vi "VI Linearisierung v2.vi"() -> ()   [LabVIEW 2020, in "Linearisierung v2.lvlib"] (continued)
                        n1066 = Concatenate Strings(w1663, "\r", w1659) -> (w1662:string)
                        n1067 = local write "Status kalibrieren"(w1662) -> ()
                      }
                    }
                  }
                  frame #1 {
                    n1068 = call "FGV-Funktionstasten.vi"("Herkunft"="Linearisierung", "Zustand"=Zustaende."Cal-Gas", "Aktion"=Funktionstasten-Aktion."Zustand setzen") -> ()  [unwired: 5 in, 8 out]
                  }
                  frame #2 {
                    n1069 = call "FID Manuell Kalibrieren.vi"("Kalibrieren"=FID_Kalibrieren."THC Nullpunkt") -> ()  [unwired: 9 in, 2 out]
                  }
                  frame #3 {
                    n1070 = call "Gasteiler_Standby.vi"() -> ()  [unwired: 12 in]
                    n1071 = call "FGV-Funktionstasten.vi"("Herkunft"="Linearisierung", "Zustand"=Zustaende."Standby", "Aktion"=Funktionstasten-Aktion."Zustand setzen") -> ()  [unwired: 5 in, 8 out]
                  }
                }
              }
              frame "PNS" {
                n1072 = flat-sequence {
                  frame #0 {
                    n1073 = call "FGV-Funktionstasten.vi"("Herkunft"="Linearisierung", "Zustand"=Zustaende."Cal-Gas", "Aktion"=Funktionstasten-Aktion."Zustand setzen") -> ()  [unwired: 5 in, 8 out]
                  }
                  frame #1 {
                    n1074 = call "FID Manuell Kalibrieren.vi"("Kalibrieren"=FID_Kalibrieren."THC Nullpunkt") -> ()  [unwired: 9 in, 2 out]
                  }
                  frame #2 {
                    n1075 = call "FGV-Funktionstasten.vi"("Herkunft"="Linearisierung", "Zustand"=Zustaende."Standby", "Aktion"=Funktionstasten-Aktion."Zustand setzen") -> ()  [unwired: 5 in, 8 out]
                  }
                }
              }
              frame "ohne Gasteiler" {
                n1076 = flat-sequence {
                  frame #0 {
                    n1077 = call "FGV-Funktionstasten.vi"("Herkunft"="Linearisierung", "Zustand"=Zustaende."0-Gas", "Aktion"=Funktionstasten-Aktion."Zustand setzen") -> ()  [unwired: 5 in, 8 out]
                  }
                  frame #1 {
                    n1078 = call "FID Manuell Kalibrieren.vi"("Kalibrieren"=FID_Kalibrieren."THC Nullpunkt") -> ()  [unwired: 9 in, 2 out]
                  }
                  frame #2 {
                    n1079 = call "FGV-Funktionstasten.vi"("Herkunft"="Linearisierung", "Zustand"=Zustaende."Standby", "Aktion"=Funktionstasten-Aktion."Zustand setzen") -> ()  [unwired: 5 in, 8 out]
                  }
                }
              }
            }
          }
        }
        n1080 = case shown="True" "PMD  E kalibrieren" {
          tunnel: w1568 -> [_ w1575]
          tunnel: w1567 -> [_ w1574]
          frame False {
          }
          frame True {
            n1081 = case shown="\"Gasteiler\", Standard" w1575 {
              tunnel: w1574 -> [w1576 _ _]
              frame "Gasteiler", Default {
                n1082 = stacked-sequence {
                  tunnel: w1576 -> [w1577 _ _ _]
                  frame #0 {
                    n1083 = local read "Anforderung"() -> (w1578:T4)
                    n1084 = case shown="False" w1578 {
                      tunnel: w1577 -> [w1579 _]
                      frame False {
                        n1085 = local read "Status kalibrieren"() -> (w1582:string)
                        n1086 = call "Texte in VIs uebersetzen.vi"("Sprachliste"=w1579, "String zum Übersetzen"="Keine Anforderung Gasteiler!\n0-Gas manuell aufschalten!" ("String")) -> ("String zum Übersetzen"=w1580:string)  [unwired: 9 in, 4 out]
                        n1087 = Concatenate Strings(w1582, "\r", w1580) -> (w1583:string)
                        n1088 = local write "Status kalibrieren"(w1583) -> ()
                      }
                      frame True {
                        n1089 = call "Gasteiler_Endpunkt.vi"() -> ()  [unwired: 12 in]
                      }
                    }
                  }
                  frame #1 {
                    n1090 = call "FGV-Funktionstasten.vi"("Herkunft"="Linearisierung", "Zustand"=Zustaende."Cal-Gas", "Aktion"=Funktionstasten-Aktion."Zustand setzen") -> ()  [unwired: 5 in, 8 out]
                  }
                  frame #2 {
                    n1091 = call "PMA Manuell Kalibrieren.vi"("GT"=TRUE, "Kalibrieren"=Kalibrierung_O2."Endpunkt O2") -> ()  [unwired: 8 in, 2 out]
                  }
                  frame #3 {
                    n1092 = call "Gasteiler_Standby.vi"() -> ()  [unwired: 12 in]
                    n1093 = call "FGV-Funktionstasten.vi"("Herkunft"="Linearisierung", "Zustand"=Zustaende."Standby", "Aktion"=Funktionstasten-Aktion."Zustand setzen") -> ()  [unwired: 5 in, 8 out]
                  }
                }
              }
              frame "PNS" {
                n1094 = flat-sequence {
                  frame #0 {
                    n1095 = call "FGV-Funktionstasten.vi"("Herkunft"="Linearisierung", "Zustand"=Zustaende."Cal-Gas", "Aktion"=Funktionstasten-Aktion."Zustand setzen") -> ()  [unwired: 5 in, 8 out]
                  }
                  frame #1 {
                    n1096 = call "PMA Manuell Kalibrieren.vi"("Kalibrieren"=Kalibrierung_O2."Endpunkt O2") -> ()  [unwired: 9 in, 2 out]
                  }
                  frame #2 {
                    n1097 = call "FGV-Funktionstasten.vi"("Herkunft"="Linearisierung", "Zustand"=Zustaende."Standby", "Aktion"=Funktionstasten-Aktion."Zustand setzen") -> ()  [unwired: 5 in, 8 out]
                  }
                }
              }
              frame "ohne Gasteiler" {
                n1098 = flat-sequence {
                  frame #0 {
                    n1099 = call "FGV-Funktionstasten.vi"("Herkunft"="Linearisierung", "Zustand"=Zustaende."0-Gas", "Aktion"=Funktionstasten-Aktion."Zustand setzen") -> ()  [unwired: 5 in, 8 out]
                  }
                  frame #1 {
                    n1100 = call "PMA Manuell Kalibrieren.vi"("GT"=TRUE, "Kalibrieren"=Kalibrierung_O2."Endpunkt O2") -> ()  [unwired: 8 in, 2 out]
                  }
                  frame #2 {
                    n1101 = call "FGV-Funktionstasten.vi"("Herkunft"="Linearisierung", "Zustand"=Zustaende."Standby", "Aktion"=Funktionstasten-Aktion."Zustand setzen") -> ()  [unwired: 5 in, 8 out]
                  }
                }
              }
            }
          }
        }
      }
      event Value Change {
        n1102 = event-data() -> ()  [unwired: 1 in, 1 out]
        n1103 = call "FGV CalGas.vi"("Aktionen"=FGV_CalGas_Aktionen."Aufschaltung CalGas", "Aufschaltung CalGas"="Aufschaltung CalGas") -> ()  [unwired: 5 in, 5 out]
      }
      event Value Change {
        w1724 = T4 TRUE  # Gasteiler Spülen
        n1104 = event-data() -> ()  [unwired: 1 in, 1 out]
        n1105 = case shown="True" "Gasteiler Spülen" {
          frame False {
          }
          frame True {
            n1106 = call "FGV Gasteiler.vi"("Aktionen"=Aktionen_FGV_Gasteiler_Daten."lesen") -> ("Gasteiler Type"=w1736:T15)  [unwired: 11 in, 7 out]
            n1107 = case shown="0, Standard" w1736 {
              frame 0, Default {
                n1108 = call "AK Komm.vi"("Aktionen"=Aktionen_AK_Komm."SRUC") -> ()  [unwired: 4 in, 7 out]
              }
            }
          }
        }
        n1109 = case shown="True" "Gasteiler EP spülen" {
          frame False {
          }
          frame True {
            n1110 = call "FGV Gasteiler.vi"("Aktionen"=Aktionen_FGV_Gasteiler_Daten."lesen") -> ("Gasteiler Type"=w1727:T15)  [unwired: 11 in, 7 out]
            n1111 = case shown="1" w1727 {
              frame 1 {
                w1729 = u32 750 ("Zu wartende ms")
                n1112 = flat-sequence {
                  tunnel: w1729 -> [w1731]
                  tunnel: w1729 -> [w1733]
                  frame #0 {
                    n1113 = call "AK Komm_ALT.vi"("Aktionen_ALT"=Aktionen_AK_Komm_ALT."SSPL") -> ()  [unwired: 6 in, 5 out]
                  }
                  frame #1 {
                    n1114 = Wait (ms)(milliseconds to wait=w1731) -> ()  [unwired: 1 out]
                  }
                  frame #2 {
                    n1115 = call "AK Komm_ALT.vi"("Aktionen_ALT"=Aktionen_AK_Komm_ALT."SSPL") -> ()  [unwired: 6 in, 5 out]
                  }
                  frame #3 {
                    n1116 = Wait (ms)(milliseconds to wait=w1733) -> ()  [unwired: 1 out]
                  }
                  frame #4 {
                    n1117 = call "AK Komm_ALT.vi"("Aktionen_ALT"=Aktionen_AK_Komm_ALT."SSPL") -> ()  [unwired: 6 in, 5 out]
                  }
                }
              }
              frame 0, Default {
                n1118 = call "AK Komm.vi"("Aktionen"=Aktionen_AK_Komm."SSPL") -> ()  [unwired: 4 in, 7 out]
              }
            }
          }
        }
      }
      event Value Change {
        n1119 = event-data() -> ()  [unwired: 1 in, 1 out]
        n1120 = call "FGV Gasteiler.vi"("Aktionen"=Aktionen_FGV_Gasteiler_Daten."lesen") -> ("Anforderung"=w1743:bool)  [unwired: 11 in, 7 out]
        n1121 = case shown="True" w1743 {
          tunnel: w1742 -> [w1745 _]
          frame False {
            n1122 = call "Texte in VIs uebersetzen.vi"("Sprachliste"=w1745, "String zum Übersetzen"="Gasteiler\nKeine Anforderung!" ("Nachricht")) -> ("String zum Übersetzen"=w1748:string)  [unwired: 9 in, 4 out]
            n1123 = call "Texte in VIs uebersetzen.vi"("Sprachliste"=w1745, "String zum Übersetzen"="OK") -> ("String zum Übersetzen"=w1747:string)  [unwired: 9 in, 4 out]
            n1124 = One Button Dialog(message=w1748, button name ("OK")=w1747) -> ()  [unwired: 1 out]
          }
          frame True {
            n1125 = call "FGV_Betreibsdaten.vi"("Gase schreiben"="Gase", "Enum"=Aktion_FGV_Betriebsdaten."Gase schreiben") -> ("error out"=w1760:errorcluster)  [unwired: 10 in, 7 out]
            n1126 = call "FGV_Kommunikation.vi"("error in"=w1760, "Aktion"=Aktion_FGV_Kom."Gase") -> ("error out"=w1756:errorcluster)  [unwired: 5 in, 4 out]
            n1127 = call "FGV_Betreibsdaten.vi"("error in (no error)"=w1756, "Enum"=Aktion_FGV_Betriebsdaten."Lesen") -> ("Gase schreiben"=w1755:T63, "Gase lesen"=w1754:T63, "error out"=w1752:errorcluster)  [unwired: 10 in, 5 out]
            n1128 = Not Equal?(x=w1755, y=w1754) -> (x != y?=w1757:T181)
            n1129 = Cluster To Array(cluster=w1757) -> (array=w1758:bool[])
            n1130 = call <vilib>:"Clear Errors.vi"("error in (no error)"=w1752) -> ()  [unwired: 5 in, 2 out]
            n1131 = Or Array Elements(Boolean array=w1758) -> (logical OR=→"Fehler Kommunikation\nGase":bool)
          }
        }
      }
      event "Vaporizer einschalten": Value Change {
        n1132 = event-data() -> ()  [unwired: 1 in, 1 out]
        n1133 = call "FGV Gasteiler.vi"("Aktionen"=Aktionen_FGV_Gasteiler_Daten."lesen") -> ("Anforderung"=w1766:bool)  [unwired: 11 in, 7 out]
        n1134 = case shown="True" w1766 {
          tunnel: w1765 -> [w1768 _]
          frame False {
            n1135 = call "Texte in VIs uebersetzen.vi"("Sprachliste"=w1768, "String zum Übersetzen"="Gasteiler\nKeine Anforderung!" ("Nachricht")) -> ("String zum Übersetzen"=w1771:string)  [unwired: 9 in, 4 out]
            n1136 = call "Texte in VIs uebersetzen.vi"("Sprachliste"=w1768, "String zum Übersetzen"="OK") -> ("String zum Übersetzen"=w1770:string)  [unwired: 9 in, 4 out]
            n1137 = One Button Dialog(message=w1771, button name ("OK")=w1770) -> ()  [unwired: 1 out]
          }
          frame True {
            n1138 = case shown="True" "Vaporizer einschalten" {
              tunnel: [w1787 w1794] -> w1778
              frame False {
                n1139 = property on="Pumpe Ein/Aus" class="Ring (strikt)"("Value"=0.0 ("Wert")) -> (error out=w1789:errorcluster)  [unwired: 2 in, 1 out]
                n1140 = property on="Solltemperatur" class="DigWert (strikt)"("Value"=0.0 ("Wert")) -> (error out=w1788:errorcluster)  [unwired: 2 in, 1 out]
                n1141 = property on="Vaporizer" class="Cluster (strikt)"("DisabledEnum"=T66."Disabled and Grayed Out" ("Deaktiviert")) -> (error out=w1790:errorcluster)  [unwired: 2 in, 1 out]
                n1142 = Merge Errors(w1790, w1789, w1788) -> (w1787:errorcluster)
              }
              frame True {
                n1143 = property on="Wasser / Reagent" class="Ring (strikt)"() -> (error out=w1797:errorcluster, "Value"=w1798:dbl)  [unwired: 2 in, 1 out]
                n1144 = case shown="0, Standard" w1798 {
                  tunnel: [w1801 w1804] -> w1796
                  tunnel: w1797 -> [w1800 w1803]
                  frame 0, Default {
                    n1145 = property on="Reagent" class="Ring (strikt)"(error in=w1800, "DisabledEnum"=T66."Disabled and Grayed Out" ("Deaktiviert")) -> (error out=w1801:errorcluster)  [unwired: 1 in, 1 out]
                  }
                  frame 1 {
                    n1146 = property on="Reagent" class="Ring (strikt)"(error in=w1803, "DisabledEnum"=T66."Enabled" ("Deaktiviert")) -> (error out=w1804:errorcluster)  [unwired: 1 in, 1 out]
                  }
                }
                n1147 = property on="Vaporizer" class="Cluster (strikt)"("DisabledEnum"=T66."Enabled" ("Deaktiviert")) -> (error out=w1795:errorcluster)  [unwired: 2 in, 1 out]
                n1148 = Merge Errors(w1795, w1796) -> (w1794:errorcluster)
              }
            }
            n1149 = call "FGV_Vaporizer.vi"("Enum"=T148."Vaporizer schreiben", "error in (no error)"=w1778, "Vaporizer schreiben"="Vaporizer") -> ("error out"=w1777:errorcluster)  [unwired: 5 in, 3 out]
            n1150 = call "FGV_Kommunikation.vi"("error in"=w1777, "Aktion"=Aktion_FGV_Kom."Vaporizer" ("Enum")) -> ("error out"=w1784:errorcluster)  [unwired: 5 in, 4 out]
            n1151 = call "FGV_Vaporizer.vi"("Enum"=T148."Lesen", "error in (no error)"=w1784) -> ("error out"=w1773:errorcluster, "Vaporizer_schreiben"=w1780:T65, "Vaporizer_lesen"=w1781:T65)  [unwired: 6 in, 1 out]
            n1152 = Not Equal?(x=w1781, y=w1780) -> (x != y?=w1782:T182)
            n1153 = Cluster To Array(cluster=w1782) -> (array=w1783:bool[])
            n1154 = call <vilib>:"Clear Errors.vi"("error in (no error)"=w1773) -> ()  [unwired: 5 in, 2 out]
            n1155 = Or Array Elements(Boolean array=w1783) -> (logical OR=→"Fehler Kommunikation\nVaporizer":bool)
          }
        }
      }
      event "Standartwerte Hovacal": Value Change {
        n1156 = event-data() -> ()  [unwired: 1 in, 1 out]
        n1157 = call "FGV Gasteiler.vi"("Aktionen"=Aktionen_FGV_Gasteiler_Daten."lesen") -> ("Anforderung"=w1810:bool)  [unwired: 11 in, 7 out]
        n1158 = case shown="True" w1810 {
          tunnel: w1809 -> [w1812 _]
          frame False {
            n1159 = call "Texte in VIs uebersetzen.vi"("Sprachliste"=w1812, "String zum Übersetzen"="Gasteiler\nKeine Anforderung!" ("Nachricht")) -> ("String zum Übersetzen"=w1815:string)  [unwired: 9 in, 4 out]
            n1160 = call "Texte in VIs uebersetzen.vi"("Sprachliste"=w1812, "String zum Übersetzen"="OK") -> ("String zum Übersetzen"=w1814:string)  [unwired: 9 in, 4 out]
            n1161 = One Button Dialog(message=w1815, button name ("OK")=w1814) -> ()  [unwired: 1 out]
          }
          frame True {
            n1162 = case shown="True" "Standartwerte Hovacal" {
              tunnel: [w1838 w1843] -> w1825
              frame True {
                w1834 = 0.0 ("Wert")
                w1832 = T66."Disabled and Grayed Out" ("Deaktiviert")
                n1163 = property on="Gesamtdurchfluss" class="DigWert (strikt)"("DisabledEnum"=w1832, "Value"=3.0 ("Wert")) -> (error out=w1837:errorcluster)  [unwired: 2 in, 1 out]
                n1164 = property on="Ausgangskonzentration\nKomponente 2" class="DigWert (strikt)"("DisabledEnum"=w1832, "Value"=w1834) -> (error out=w1835:errorcluster)  [unwired: 2 in, 1 out]
                n1165 = property on="Eingangskonzentration \nKomponente 2" class="DigWert (strikt)"("DisabledEnum"=w1832, "Value"=w1834) -> (error out=w1836:errorcluster)  [unwired: 2 in, 1 out]
                n1166 = property on="Eingangskonzentration \nTrägergas" class="DigWert (strikt)"("DisabledEnum"=w1832, "Value"=100.0 ("Wert")) -> ()  [unwired: 2 in, 2 out]
                n1167 = Merge Errors(w1837, w1836, w1835) -> (w1838:errorcluster)
              }
              frame False {
                w1839 = T66."Enabled" ("Deaktiviert")
                n1168 = property on="Gesamtdurchfluss" class="DigWert (strikt)"("DisabledEnum"=w1839) -> (error out=w1842:errorcluster)  [unwired: 2 in, 1 out]
                n1169 = property on="Eingangskonzentration \nKomponente 2" class="DigWert (strikt)"("DisabledEnum"=w1839) -> (error out=w1841:errorcluster)  [unwired: 2 in, 1 out]
                n1170 = property on="Ausgangskonzentration\nKomponente 2" class="DigWert (strikt)"("DisabledEnum"=w1839) -> (error out=w1840:errorcluster)  [unwired: 2 in, 1 out]
                n1171 = Merge Errors(w1842, w1841, w1840) -> (w1843:errorcluster)
              }
            }
            n1172 = call "FGV_Betreibsdaten.vi"("Sollwert schreiben"="Daten", "error in (no error)"=w1825, "Enum"=Aktion_FGV_Betriebsdaten."Sollwerte schreiben" ("Aktion")) -> ("error out"=w1824:errorcluster)  [unwired: 9 in, 7 out]
            n1173 = call "FGV_Kommunikation.vi"("error in"=w1824, "Aktion"=Aktion_FGV_Kom."Betriebsparameter" ("Enum")) -> ("error out"=w1821:errorcluster)  [unwired: 5 in, 4 out]
            n1174 = call "FGV_Betreibsdaten.vi"("error in (no error)"=w1821, "Enum"=Aktion_FGV_Betriebsdaten."Lesen" ("Aktion")) -> ("Sollwerte lesen"=w1829:T64, "Sollwert für Vergleich"=w1828:T64, "error out"=w1819:errorcluster)  [unwired: 10 in, 5 out]
            n1175 = Not Equal?(x=w1829, y=w1828) -> (x != y?=w1826:T183)
            n1176 = call <vilib>:"Clear Errors.vi"("error in (no error)"=w1819) -> ()  [unwired: 5 in, 2 out]
            n1177 = Cluster To Array(cluster=w1826) -> (array=w1827:bool[])
            n1178 = Or Array Elements(Boolean array=w1827) -> (logical OR=→"Fehler Kommunikaton\nBetriebsdaten":bool)
          }
        }
      }
      event Value Change {
        n1179 = event-data() -> ()  [unwired: 1 in, 1 out]
        n1180 = call "Genauigkeit Polynom 2 String.vi"() -> ("Format-String Polynom 2 Sting"=w1845:string)  [unwired: 9 in, 2 out]
        n1181 = for {
          tunnel: "PolynomTabelleEingabe" -> [w1856] mode=indexing
          tunnel: [w1855] -> w1847 mode=indexing
          tunnel: w1845 -> [w1854]
          # "#PolynomDBL"
          n1182 = for {
            tunnel: w1856 -> [w1860] mode=indexing
            tunnel: [w1859] -> w1855 mode=indexing
            tunnel: w1854 -> [w1857]
            n1183 = Scan Value(string=w1860, format string=w1857, default (0 dbl)=0.0) -> (value=w1859:dbl)  [unwired: 1 out]
          }
        }
        n1184 = call "Polynom Daten speichern.vi"("Aktionen"=Aktionen_Polynom_Daten_speichern."schreiben alle", "Aktiv"="PolynomAktiv", "Polynome"=w1847) -> ("Polynome"=w1853:dbl[][])  [unwired: 3 in, 5 out]
        n1185 = call "Polynom Daten speichern.vi"("Aktionen"=Aktionen_Polynom_Daten_speichern."speichern", "Polynome"=w1853) -> ()  [unwired: 4 in, 6 out]
      }
      event "Hauptregisterkarte": Value Change {
        n1186 = event-data() -> ()  [unwired: 1 in, 1 out]
        n1187 = call "Komponentenausgabe.vi"() -> ("Gaskomponente"=w1865:T7)  [unwired: 8 in, 3 out]
        n1188 = call "Einheiten finden.vi"("Komponente"=w1865) -> ("Einheit in String"=w1864:string)  [unwired: 6 in, 4 out]
        n1189 = case shown="\"LIN Anpassung\"" "Hauptregisterkarte" {
          tunnel: w1865 -> [_ _ w1918 w1966 _ _ _ _ _ _]
          tunnel: [_ _ _ _ _ _ _ TRUE _ _] -> w1869
          tunnel: w1868 -> [_ w1887 _ _ _ _ _ _ _ _]
          tunnel: w1864 -> [_ _ w1928 w1985 _ _ _ _ _ _]
          tunnel: w1867 -> [_ _ _ w1986 _ _ _ _ _ _]
          tunnel: w1866 -> [_ w1886 w1927 _ _ _ _ _ _ _]
          tunnel: w1862 -> [_ _ _ _ _ _ _ _ _ w2030]
          tunnel: w1861 -> [_ _ _ _ _ _ _ _ _ w2029]
          frame "Einstellungen", Default {
          }
          frame "Daten aufzeichnen" {
            # "#LinEinheiten #HovaCALMultiMFC"
            n1190 = local read "passive Komponente:"() -> (w1882:u16)
            n1191 = local read "Gasnummer Generieren"() -> (w1874:T49)
            n1192 = Equal To 0?(x=w1882) -> (x = 0?=w1884:bool)
            n1193 = Decrement(x=w1882) -> (x-1=w1883:u16)
            n1194 = call "Komponentenausgabe HovaCAL fix.vi"("Gasnummer in"=w1874) -> ("Gaskomponente"=w1880:T7)  [unwired: 7 in, 3 out]
            n1195 = Select(t=w1880, s=w1884, f=w1883) -> (s? t:f=w1879:T7)
            n1196 = call "Einheiten finden.vi"("Komponente"=w1879) -> ("Einheit in String"=w1881:string)  [unwired: 6 in, 4 out]
            n1197 = call "Lin Daten aufarbeiten.vi"("Index (Seite)"=w1879, "Aktionen"=Aktion_Lin_Daten_aufarbeiten."lesen") -> ("Eingabetabelle"=w1890:T54, "Lin-Polynom"=w1878:T119)  [unwired: 15 in, 9 out]
            n1198 = disable-structure shown="Aktiviert" {
              disable-tunnel: w1879 -> [w1895 w1900]
              disable-tunnel: w1878 -> [w1894 w1901]
              disable-tunnel: [w1893 w1903] -> w1877
              disable-tunnel: [w1892 w1902] -> w1876
              disable-tunnel: [_ w1904] -> w1875
              frame Disabled {
                n1199 = call "Get Autorange Bereiche.vi"("Gaskomponente"=w1895) -> ("error out"=w1896:errorcluster, "Autorange Bereiche"=w1899:T7[])  [unwired: 8 in, 1 out]
                n1200 = call "Set Spanfactors and Offests in Lin-Protocol.vi"("Lin-Polynom"=w1894) -> ("Offset"=w1897:sgl[], "Span"=w1898:sgl[])  [unwired: 7 in, 2 out]
                n1201 = call "Get Autorange Spanfactors and Offsets.vi"("error in (no error)"=w1896, "Autorange Bereiche"=w1899, "Offset"=w1897, "Span"=w1898) -> ("Autorange Offsets"=w1892:string, "Autorange Spanfactors"=w1893:string)  [unwired: 3 in, 3 out]
              }
              frame Enabled {
                # "#PDF_manu_MG"
                n1202 = call "Component Get Daten aufzeichnen.vi"("Lin-Polynom"=w1901, "Gaskomponente"=w1900) -> ("Autorange Offsets"=w1902:string, "Autorange Spanfactors"=w1903:string, "Polynome"=w1904:T184)  [unwired: 6 in, 1 out]
              }
            }
            n1203 = call "Einheiten in Tabellenspalten.vi"("Einheit"=w1881, "Tabelle (Eingang)"=w1887) -> ("Einheit out"=w1885:string)  [unwired: 7 in, 2 out]
            n1204 = local write "Einheit"(w1881) -> ()
            n1205 = local write "Einheit Deviation"(w1881) -> ()
            n1206 = call "AusgabeTabelle zusammenbauen.vi"("Eingabetabelle"=w1890) -> ("Eingabetabelle behandelt"=w1888:string[][], "Ausgabetabelle"=→"Ausgabetabelle":T53)  [unwired: 8 in, 1 out]
            n1207 = call "Einheiten in Tabellenspalten.vi"("Einheit"=w1885, "Tabelle (Eingang)"=w1886) -> ()  [unwired: 7 in, 3 out]
            n1208 = local write "Eingabetabelle"(w1888) -> ()
            n1209 = local write "Polynom"(w1875) -> ()
            n1210 = local write "Spanfactor"(w1877) -> ()
            n1211 = local write "Offset"(w1876) -> ()
          }
          frame "EPA 1065-307" {
            # "#PDF_manu_MG"
            # "#LinEinheiten"
            n1212 = local read "Gasnummer EPA"() -> (w1925:T49)
            n1213 = call "Einheiten in Tabellenspalten.vi"("Einheit"=w1928, "Tabelle (Eingang)"=w1927) -> ()  [unwired: 7 in, 3 out]
            n1214 = call "aktueller SPAN und Komponent Index.vi"() -> ("akt SPAN out"=w1913:i32)  [unwired: 7 in, 4 out]
            n1215 = Decrement(x=w1925) -> (x-1=w1909:T49)
            n1216 = local read "EPA Filename override"() -> (w1907:T1)
            n1217 = Bundle("akt SPAN out"=w1913, w1909) -> (w1912:cluster{"akt SPAN out":i32, T49})  [unwired: 1 in]
            n1218 = call "EPA Polynom Ordnung je Komponente für Protokoll.vi"("Aktion"=Aktion_EPA_Polynom_Ordnung_je_Komponente_für_Protokoll."lesen", "Index in"=w1912) -> ("EPA Optionsfeld out"=w1914:T2)  [unwired: 5 in, 3 out]
            n1219 = call "Lin Daten aufarbeiten.vi"("Index (Seite)"=w1918, "Aktionen"=Aktion_Lin_Daten_aufarbeiten."lesen") -> ("Index (Seite) out"=w1921:i32, "Lin-Polynom"=w1919:T119, "error out"=w1920:errorcluster)  [unwired: 15 in, 8 out]
            n1220 = Bundle By Name(cluster=w1919, "EPA Optionsfeld"=w1914) -> (w1923:T119)
            n1221 = call "FGV SPAN Verriegelung.vi"("aktion"=Aktion_FGV_SPAN_Verriegelung."lesen") -> ("locked"=w1910:bool)  [unwired: 8 in, 2 out]
            n1222 = local write "EPA Optionsfeld"(w1914) -> ()
            n1223 = Not(x=w1907) -> (.not. x?=w1906:T1)
            n1224 = Not(x=w1910) -> (.not. x?=w1905:bool)
            n1225 = call "Lin Daten aufarbeiten.vi"("Index (Seite)"=w1921, "Lin-Polynom"=w1923, "error in (no error)"=w1920, "Aktionen"=Aktion_Lin_Daten_aufarbeiten."Protkolldaten") -> ("Index (Seite) out"=w1917:i32, "error out"=w1915:errorcluster)  [unwired: 13 in, 9 out]
            n1226 = And(x=w1906, y=w1905) -> (x .and. y?=w1908:T1)
            n1227 = case shown="True" w1908 {
              tunnel: w1917 -> [_ w1944]
              tunnel: w1909 -> [_ w1943]
              frame False {
              }
              frame True {
                # "#Lin_Load_Polynom_Question"
                n1228 = disable-structure shown="Aktiviert" {
                  disable-tunnel: [w1949 w1955] -> w1946
                  disable-tunnel: [w1948 w1954] -> w1945
                  disable-tunnel: w1944 -> [w1947 _]
                  disable-tunnel: w1943 -> [_ w1953]
                  frame Disabled {
                    n1229 = call "FGV Gasliste.vi"("Aktionen"=FGV_FT-IR_Gasliste_Aktionen."lesen") -> ("Aktuelle Gasliste gesamt"=w1951:T48[])  [unwired: 8 in, 2 out]
                    n1230 = Index Array(array=w1951, index=w1947) -> (element=w1950:T48)
                    n1231 = call "Namen fuer File erzeugen.vi"("String Eingabe"=w1950) -> ("File Name LIN"=w1948:string, "File Name EPA"=w1949:string)  [unwired: 9 in]
                  }
                  frame Enabled {
                    n1232 = call "MG FileName.vi"("Gasnummer:"=w1953) -> ("LIN TXT Datei Name"=w1954:string, "EPA TXT Datei Name"=w1955:string)  [unwired: 7 in, 2 out]
                  }
                }
                n1233 = local write "EPA Filename"(w1946) -> ()
                n1234 = local write "File Name LIN"(w1945) -> ()
              }
            }
            n1235 = control-ref of="EPA Auswertung"() -> (w1929:refnum<vi>)
            n1236 = call "Lin Daten aufarbeiten.vi"("Index (Seite)"=w1917, "error in (no error)"=w1915, "Aktionen"=Aktion_Lin_Daten_aufarbeiten."EPA auswerten") -> ("Index (Seite) out"=w1916:i32, "error out"=w1940:errorcluster)  [unwired: 14 in, 9 out]
            n1237 = call "Lin Daten aufarbeiten.vi"("Index (Seite)"=w1916, "error in (no error)"=w1940, "Aktionen"=Aktion_Lin_Daten_aufarbeiten."lesen") -> ("Aktiv EPA"=w1932:T57, "Eingabetabelle"=w1937:T54, "EPA Auswertung"=w1931:cluster{sgl[], sgl[], bool[]}, "error out"=w1939:errorcluster)  [unwired: 14 in, 7 out]
            n1238 = call "EPA_Tabelle zusammenbauen.vi"("error in (no error)"=w1939, "Eingabetabelle"=w1937) -> ("error out"=w1935:errorcluster, "XY-Graph"=→"XY-Graph EPA":cluster{dbl[], dbl[]}[], "EPA Ausgabetabelle"=→"EPA Ausgabetabelle":string[][])  [unwired: 7 in]
            n1239 = local write "Aktiv"(w1932) -> ()
            n1240 = Unbundle(w1931) -> (w1930:bool[])  [unwired: 2 out]
            n1241 = call "FGV Auswertung sammeln.vi"("Aktion"=Aktion_FGV_Auswertung_sammeln."lesen", "error in (no error)"=w1935) -> ("LINVer Auswertung"=→"EPA Auswertung":string[][])  [unwired: 7 in, 2 out]
            n1242 = call "Zellen einfaerben.vi"("Färben"=w1930, "Tabellenref."=w1929) -> ()  [unwired: 10 in]
          }
          frame "LIN Anpassung" {
            # "#PDF_manu_MG"
            # "#LinEinheiten #AutorangeSpanfactorsOffsets"
            n1243 = local read "Gasnummer LIN"() -> (w1971:T49)
            n1244 = call "Einheiten in Tabellenspalten.vi"("Einheit"=w1985, "Tabelle (Eingang)"=w1986) -> ()  [unwired: 7 in, 3 out]
            n1245 = call "aktueller SPAN und Komponent Index.vi"() -> ("akt SPAN out"=w1967:i32)  [unwired: 7 in, 4 out]
            n1246 = Decrement(x=w1971) -> (x-1=w1960:T49)
            n1247 = Bundle("akt SPAN out"=w1967, w1960) -> (w1968:cluster{"akt SPAN out":i32, T49})  [unwired: 1 in]
            n1248 = local read "LIN Filename override"() -> (w1958:T1)
            n1249 = call "LIN Polynom Ordnung je Komponente für Protokoll.vi"("Aktion"=Aktion_LIN_Polynom_Ordnung_je_Komponente_für_Protokoll."lesen", "Index in"=w1968) -> ("Polynom-Ordnung view only out"=w1969:T55)  [unwired: 3 in, 6 out]
            n1250 = local write "Polynom-Ordnung"(w1969) -> ()
            n1251 = call "FGV SPAN Verriegelung.vi"("aktion"=Aktion_FGV_SPAN_Verriegelung."lesen") -> ("locked"=w1961:bool)  [unwired: 8 in, 2 out]
            n1252 = call "Lin Daten aufarbeiten.vi"("Index (Seite)"=w1966, "Polynom-Ordnung"=w1969, "Aktionen"=Aktion_Lin_Daten_aufarbeiten."Lin auswerten") -> ("Index (Seite) out"=w1964:i32, "error out"=w1987:errorcluster)  [unwired: 14 in, 9 out]
            n1253 = call "Get Autorange Bereiche.vi"("Gaskomponente"=w1966) -> ("error out"=w1977:errorcluster, "Autorange Bereiche"=w1984:T7[])  [unwired: 8 in, 1 out]
            n1254 = Not(x=w1961) -> (.not. x?=w1956:bool)
            n1255 = Not(x=w1958) -> (.not. x?=w1957:T1)
            n1256 = call "Lin Daten aufarbeiten.vi"("Index (Seite)"=w1964, "error in (no error)"=w1987, "Aktionen"=Aktion_Lin_Daten_aufarbeiten."lesen") -> ("Aktiv LIN"=w1989:bool[], "Eingabetabelle"=w1993:T54, "Index (Seite) out"=w1963:i32, "Lin-Polynom"=w1965:T119, "error out"=w1982:errorcluster)  [unwired: 14 in, 6 out]
            n1257 = And(x=w1957, y=w1956) -> (x .and. y?=w1959:T1)
            n1258 = call "Set Spanfactors and Offests in Lin-Protocol.vi"("error in (no error)"=w1982, "Lin-Polynom"=w1965) -> ("error out"=w1981:errorcluster, "Offset"=w1978:sgl[], "Span"=w1979:sgl[], "Lin-Polynom out"=w1980:T119)  [unwired: 6 in]
            n1259 = case shown="True" w1959 {
              tunnel: w1963 -> [_ w1995]
              tunnel: w1960 -> [_ w1994]
              frame False {
              }
              frame True {
                # "#Lin_Load_Polynom_Question"
                n1260 = disable-structure shown="Aktiviert" {
                  disable-tunnel: [w2000 w2006] -> w1997
                  disable-tunnel: [w1999 w2005] -> w1996
                  disable-tunnel: w1995 -> [w1998 _]
                  disable-tunnel: w1994 -> [_ w2004]
                  frame Disabled {
                    n1261 = call "FGV Gasliste.vi"("Aktionen"=FGV_FT-IR_Gasliste_Aktionen."lesen") -> ("Aktuelle Gasliste gesamt"=w2002:T48[])  [unwired: 8 in, 2 out]
                    n1262 = Index Array(array=w2002, index=w1998) -> (element=w2001:T48)
                    n1263 = call "Namen fuer File erzeugen.vi"("String Eingabe"=w2001) -> ("File Name LIN"=w1999:string, "File Name EPA"=w2000:string)  [unwired: 9 in]
                  }
                  frame Enabled {
                    n1264 = call "MG FileName.vi"("Gasnummer:"=w2004) -> ("LIN TXT Datei Name"=w2005:string, "EPA TXT Datei Name"=w2006:string)  [unwired: 7 in, 2 out]
                  }
                }
                n1265 = local write "EPA Filename"(w1997) -> ()
                n1266 = local write "File Name LIN"(w1996) -> ()
              }
            }
            n1267 = call "LinTabelle zusammenbauen.vi"("error in (no error)"=w1982, "Eingabetabelle"=w1993) -> ("XY-Graph"=→"XY-Graph LIN":cluster{dbl[], dbl[]}[], "LIN Ausgabetabelle"=→"LIN Ausgabetabelle":string[][])  [unwired: 6 in, 2 out]
            n1268 = call "Lin Daten aufarbeiten.vi"("Index (Seite)"=w1963, "Lin-Polynom"=w1980, "error in (no error)"=w1981, "Aktionen"=Aktion_Lin_Daten_aufarbeiten."Protkolldaten") -> ("Lin-Polynom"=w1974:T119)  [unwired: 13 in, 10 out]
            n1269 = local write "Aktiv LIN"(w1989) -> ()
            n1270 = Unbundle By Name(w1974) -> ("Polynomkoeff."=w1976:dbl[])
            n1271 = call "Get Autorange Spanfactors and Offsets.vi"("error in (no error)"=w1977, "Autorange Bereiche"=w1984, "Offset"=w1978, "Span"=w1979) -> ("Autorange Offsets"=w1972:string, "Autorange Spanfactors"=w1973:string)  [unwired: 3 in, 3 out]
            n1272 = Array To Cluster(array=w1976) -> (cluster=w1975:T185)
            n1273 = local write "LIN Polynomkoeffizienten"(w1975) -> ()
            n1274 = local write "Spanfactor LIN"(w1973) -> ()
            n1275 = local write "Offset LIN"(w1972) -> ()
          }
          frame "Polynomkoeffizienten" {
            n1276 = call "Polynom Daten speichern.vi"("Aktionen"=Aktionen_Polynom_Daten_speichern."lesen") -> ("Aktiv"=w2009:bool[], "Polynome"=w2008:dbl[][])  [unwired: 5 in, 4 out]
            n1277 = call "Genauigkeit Polynom 2 String.vi"() -> ("Format-String Polynom 2 Sting"=w2007:string)  [unwired: 9 in, 2 out]
            n1278 = for {
              tunnel: w2008 -> [w2014] mode=indexing
              tunnel: [w2013] -> w2010 mode=indexing
              tunnel: w2007 -> [w2012]
              # "#PolynomDBL"
              n1279 = for {
                tunnel: w2014 -> [w2017] mode=indexing
                tunnel: [w2016] -> w2013 mode=indexing
                tunnel: w2012 -> [w2015]
                n1280 = Format Value(format string=w2015, value (0)=w2017) -> (output string=w2016:string)  [unwired: 1 in]
              }
            }
            n1281 = local write "PolynomAktiv"(w2009) -> ()
            n1282 = local write "PolynomTabelleEingabe"(w2010) -> ()
          }
          frame "HovaCal Einstellungen" {
          }
          frame "HovaCAL Interface" {
            n1283 = call "FGV_HovaCAL_Interface_GetData.vi"("first flags in"=T151 {"first contact in"=TRUE, "first actual values in "=TRUE}, "Aktion"=Aktion_FGV_HovaCAL_Interface_GetData."first contact") -> ()  [unwired: 5 in, 5 out]
          }
          frame "Spanfaktor" {
            n1284 = call "Spantabellenanzeige.vi"() -> ("SpanTabelle"=w2022:T48[][])  [unwired: 10 in, 1 out]
            n1285 = Delete From Array(array=w2022, length=3 ("Länge"), index (col)=0 ("Deaktivierter Index (Spalte)")) -> (deleted portion=w2020:T48[][], array with subset deleted=w2021:T48[][])  [unwired: 1 in]
            n1286 = local write "SpanTabelleEingabe"(w2021) -> ()
            n1287 = local write "SpanTabelleAnzeige"(w2020) -> ()
          }
          frame "Kalibrierung" {
          }
          frame "Span Einstellungen" {
            n1288 = call "Span Register setzen.vi"("GD Span Eingänge"=w2030, "automatisch Boolesch (Eingang)"=w2029) -> ()  [unwired: 3 in, 7 out]
            n1289 = call "FGV SpanEinstellungen.vi"("Aktion"=Aktion_FGV_SpanEinstellungen."lesen") -> ("SpanInletClusterArray out"=w2027:T19[])  [unwired: 6 in, 4 out]
            n1290 = Index Array(array=w2027) -> (element=w2026:T19)  [unwired: 1 in]
            n1291 = local write "Span 1"(w2026) -> ()
          }
        }
        n1292 = call "FGV Span.vi"("Aktion"=Aktion_FGV_Span."Seite aktiv", "Aktiv"=w1869) -> ()  [unwired: 6 in, 4 out]
      }
      event Value Change {
        # "#LinV2_auto_singleSave"
        # "#LinV2_auto_singleSave :\n\nEPA redirect auch im auto modus wenn post processing\n\nLIN redirect flag setzen um manuell von auto all zu unterscheiden - \nAchtung, Eigenschaftsknopten in SubVIs über Referenzen (abbruch etc.) \n\noverrule PDF start, kein next, immer close - druch PDF singel pages ?!\n\nnur in automaitc + postprocessing + NOT Postprocessing PDF \n\nTesten und wahnsinnig werden ..."
        # "#Option10xSpanAuto #PDF_Interface #LinV2_auto_singleSave"
        n1293 = event-data() -> ()  [unwired: 1 in, 1 out]
        n1294 = call "FGV SpanEinstellungen.vi"("Aktion"=Aktion_FGV_SpanEinstellungen."lesen") -> ("automatisch out"=w2071:T20, "SpanInletClusterArray out"=w2072:T19[], "Punkte umkehren und PDF Optionen Cluster"=w2061:T109)  [unwired: 6 in, 2 out]
        n1295 = call "get SPAN Table.vi"("automatisch in"=w2071, "SpanInletClusterArray in"=w2072) -> ("automatisch out"=w2070:T20, "SpanInletClusterArray out"=w2058:T19[], "SpanComponentInfos-Cluster"=w2069:T186)  [unwired: 3 in, 4 out]
        n1296 = call "FGV SPAN Verriegelung.vi"("aktion"=Aktion_FGV_SPAN_Verriegelung."lesen") -> ("Flags Cluster"=w2046:T188)  [unwired: 8 in, 2 out]
        n1297 = Unbundle By Name(w2046) -> ("Save EPA redirect"=w2038:bool, "Postprocessing PDF"=w2041:bool)
        n1298 = case shown="True" w2070 {
          selector: w2070 -> [w2118 _]
          tunnel: w2058 -> [w2114 w2148]
          tunnel: [w2108 w2138] -> w2082
          tunnel: [w2102 w2144] -> w2057
          tunnel: [w2117 w2149] -> w2081
          tunnel: [w2099 w2147] -> w2080
          tunnel: [_ w2142] -> _
          tunnel: [_ w2146] -> _
          tunnel: [w2119 w2141] -> w2077
          tunnel: [w2098 w2133] -> w2051
          tunnel: [w2109 w2136] -> w2073
          tunnel: [w2118 w2145] -> w2068
          tunnel: [_ w2130] -> w2065
          tunnel: [w2115 _] -> w2063
          tunnel: [w2113 _] -> w2062
          tunnel: w2061 -> [w2111 w2140]
          tunnel: [w2107 w2135] -> w2060
          tunnel: w2059 -> [w2106 w2134]
          tunnel: [w2098 w2133] -> w2053
          tunnel: [w2097 w2132] -> w2052
          tunnel: [w2094 "Pfad Auto Lin"] -> w2050
          tunnel: w2038 -> [w2088 w2123]
          tunnel: [w2091 w2125] -> w2042
          tunnel: [_ w2130] -> w2040
          tunnel: [_ w2124] -> w2032
          tunnel: [w2087 w2122] -> w2031
          frame False {
            w2119 = TRUE  # PDF start
            # "manuell"
            n1299 = local read "EPA Filename override"() -> (w2090:T1)
            n1300 = local read "LIN Filename override"() -> (w2089:T1)
            n1301 = Unbundle By Name(w2111) -> ("PDF Optionen"=w2110:T108)
            n1302 = call "get SPAN first active component.vi"("SPAN Idx"=0 ("Index out"), "SpanInletClusterArray in"=w2114) -> ("first aktive Komponente"=w2115:i32, "SPAN Idx out"=w2113:i32, "SpanInletClusterArray out"=w2112:T19[])  [unwired: 6 in, 1 out]
            n1303 = local read "EPA Filename"() -> (w2092:T12)
            n1304 = local read "EPA Pfad"() -> (w2095:T9)
            n1305 = call "get SPAN active components count.vi"("SPAN Idx"=w2113, "SpanInletClusterArray in"=w2112) -> ("error out"=w2103:errorcluster, "Anzahl aktive Komponenten"=w2101:i32, "SPAN Idx out"=w2104:i32, "SpanInletClusterArray out"=w2105:T19[])  [unwired: 6 in]
            n1306 = call "get SPAN all component names.vi"("error in (no error)"=w2103, "Anzahl aktive Komponenten"=w2101, "active SPAN Idx"=w2104, "SpanInletClusterArray in"=w2105) -> ("Anzahl aktive Komponenten out"=w2100:i32, "SpanInletClusterArray out"=w2102:T19[], "Component Infos"=w2099:T187)  [unwired: 1 in, 4 out]
            n1307 = Get Date/Time In Seconds() -> (seconds since 1Jan1904=w2117:timestamp)
            n1308 = Select(t=w2095, s=w2088, f="Pfad LIN") -> (s? t:f=w2094:T9)
            n1309 = Select(t=w2090, s=w2088, f=w2089) -> (s? t:f=w2087:T1)
            n1310 = Select(t=w2092, s=w2088, f="File Name LIN") -> (s? t:f=w2091:T12)
            n1311 = call "PDF Optionen automatisch.vi"("PDF Optionen Referenzen Cluster"=w2106, "Anzahl aktive Komponenten"=w2100, "PDF Optionen (Eingang)"=w2110) -> ("Anzahl aktive Komponenten out"=w2108:i32, "PDF Optionen (Ausgang)"=w2109:T108, "PDF Einzelseiten Span"=w2098:bool, "PDF öffnen"=w2107:bool, "PDF Einzelseiten Komponenten"=w2097:bool)  [unwired: 2 in, 2 out]
          }
          frame True {
            # "#PDF_manu_MG"
            # "automatisch"
            n1312 = local read "File Name LIN"() -> (w2128:T12)
            n1313 = local read "EPA Filename"() -> (w2129:T12)
            n1314 = local read "EPA Filename override"() -> (w2121:T1)
            n1315 = local read "LIN Filename override"() -> (w2120:T1)
            n1316 = call "SPAN LIN speichern Parameter bestimmern.vi"("SpanInletClusterArray out (Eingang)"=w2148) -> ("Anzahl Komponenten OK"=w2142:bool, "gültige aktiver auto SPAN Index"=w2143:bool, "Anzahl aktive Komponenten out"=w2139:i32, "SpanInletClusterArray out (Ausgang)"=w2144:T19[], "Zeitstempel"=w2149:timestamp, "Anzahl Namen"=w2146:i32, "Component Infos"=w2147:T187, "postprocess"=w2130:bool, "PDF start"=w2141:bool)  [unwired: 2 in]
            n1317 = local read "EPA Pfad"() -> (w2127:T9)
            n1318 = local read "Pfad LIN"() -> (w2126:T9)
            n1319 = Unbundle By Name(w2140) -> ("PDF Optionen"=w2137:T108)
            n1320 = Not(x=w2143) -> (.not. x?=w2145:bool)
            n1321 = Select(t=w2127, s=w2123, f=w2126) -> (s? t:f=w2124:T9)
            n1322 = Select(t=w2121, s=w2123, f=w2120) -> (s? t:f=w2122:T1)
            n1323 = Select(t=w2129, s=w2123, f=w2128) -> (s? t:f=w2125:T12)
            n1324 = call "PDF Optionen automatisch.vi"("PDF Optionen Referenzen Cluster"=w2134, "Anzahl aktive Komponenten"=w2139, "PDF Optionen (Eingang)"=w2137) -> ("Anzahl aktive Komponenten out"=w2138:i32, "PDF Optionen (Ausgang)"=w2136:T108, "PDF Einzelseiten Span"=w2133:bool, "PDF öffnen"=w2135:bool, "PDF Einzelseiten Komponenten"=w2132:bool)  [unwired: 2 in, 2 out]
          }
        }
        n1325 = Not(x=w2041) -> (.not. x?=w2033:bool)
        n1326 = And(x=w2040, y=w2033) -> (x .and. y?=w2037:bool)
        n1327 = local write "Speichern LIN"(T4 FALSE ("Speichern LIN")) -> ()
        n1328 = Or(x=w2051, y=w2037) -> (x .or. y?=w2039:bool)
        n1329 = Not(x=w2065) -> (.not. x?=w2066:bool)
        n1330 = for {
          N: w2082 -> [_]
          tunnel: w2068 -> [w2163]
          tunnel: w2057 -> [w2220]
          tunnel: w2081 -> [w2219]
          tunnel: [w2165] -> w2074
          tunnel: w2080 -> [w2218]
          tunnel: w2079 -> [w2217]
          tunnel: w2077 -> [w2178]
          tunnel: [w2213] -> w2076
          tunnel: [w2212] -> w2075
          tunnel: w2073 -> [w2183]
          tunnel: w2069 -> [w2182]
          tunnel: [w2207] -> w2067
          tunnel: w2066 -> [w2204]
          tunnel: w2065 -> [w2203]
          shift-right: [w2200] -> _
          shift-left: w2063 -> [w2202]
          tunnel: w2062 -> [w2201]
          tunnel: w2056 -> [w2186]
          tunnel: w2055 -> [w2185]
          tunnel: w2054 -> [w2184]
          tunnel: w2053 -> [w2180]
          tunnel: w2052 -> [w2179]
          tunnel: w2039 -> [w2174]
          tunnel: w2050 -> [w2172]
          tunnel: w2049 -> [w2171]
          tunnel: [w2162] -> w2048
          tunnel: w2047 -> [w2161]
          tunnel: w2038 -> [w2160]
          tunnel: [w2158] -> w2044
          tunnel: [w2158] -> w2043
          tunnel: w2042 -> [w2157]
          tunnel: w2037 -> [w2155]
          tunnel: w2032 -> [w2151]
          tunnel: w2031 -> [w2150]
          i -> [w2187]
          # "#PDF_manu_MG #EPA_Save_redirect"
          n1331 = Equal To 0?(x=w2187) -> (x = 0?=w2176:bool)
          n1332 = case shown="True" w2163 {
            tunnel: [w2280 w2341] -> w2209
            tunnel: [w2234 w2296] -> w2164
            tunnel: w2220 -> [w2284 w2352]
            tunnel: [w2259 w2332] -> _
            tunnel: [w2258 w2331] -> w2206
            tunnel: w2219 -> [w2283 w2338]
            tunnel: w2176 -> [w2251 w2346]
            tunnel: w2218 -> [w2249 w2345]
            tunnel: w2217 -> [w2252 w2344]
            tunnel: [w2241 w2343] -> w2211
            tunnel: [w2281 w2334] -> _
            tunnel: [w2279 w2340] -> w2208
            tunnel: w2203 -> [_ w2327]
            tunnel: w2202 -> [w2237 _]
            tunnel: w2201 -> [w2236 _]
            tunnel: [w2259 _] -> w2200
            tunnel: w2186 -> [w2272 w2330]
            tunnel: w2185 -> [w2273 w2329]
            tunnel: w2184 -> [w2274 w2328]
            tunnel: [w2261 w2326] -> w2199
            tunnel: [w2260 w2325] -> w2198
            tunnel: [w2263 w2324] -> w2197
            tunnel: [w2262 w2323] -> w2196
            tunnel: [w2267 w2322] -> w2195
            tunnel: [w2266 w2321] -> w2193
            tunnel: [w2265 w2313] -> w2194
            tunnel: [w2269 w2320] -> w2191
            tunnel: [w2270 w2319] -> w2192
            tunnel: [w2268 w2318] -> w2190
            tunnel: w2183 -> [w2253 w2317]
            tunnel: [w2239 w2299] -> w2188
            tunnel: w2182 -> [w2243 w2311]
            tunnel: [w2243 w2309] -> w2181
            tunnel: w2180 -> [_ w2308]
            tunnel: w2176 -> [w2242 w2306]
            tunnel: w2172 -> [w2232 w2304]
            tunnel: [w2233 w2302] -> w2159
            tunnel: w2163 -> [_ w2295]
            tunnel: [_ w2294] -> w2162
            tunnel: w2157 -> [w2231 w2293]
            tunnel: w2151 -> [_ w2292]
            tunnel: w2150 -> [w2230 w2291]
            frame False {
              w2275 = TRUE  # postprocess
              # "manuell"
              n1333 = Increment(x=w2237) -> (x+1=w2255:i32)
              n1334 = call "get Polynom and EPA Auswahl from SPAN and Comp Index.vi"("Component Index"=w2237, "SPAN Idx"=w2236) -> ("Index Cluster"=w2235:T189, "EPA Optionsfeld out"=w2238:T2, "Polynom-Ordnung out"=w2239:T55)  [unwired: 7 in]
              n1335 = call "Set SPAN Component.vi"("Protocol_only"=TRUE, "Gasnummer"=w2255, "Autolin Hovacal (alt)"=w2272, "Daten Hovacal (alt)"=w2273) -> ("error out"=w2276:errorcluster, "Gaskomponente"=w2245:T7, "LogInfo-Einstellung-Cluster"=w2250:T190, "Komponente"=w2256:string, "Einheit in String"=w2254:string)  [unwired: 3 in]
              n1336 = Bundle("Komponente"=w2256, w2255, "Einheit in String"=w2254) -> (w2247:T191)  [unwired: 1 in]
              n1337 = Bundle("PDF Optionen (Ausgang)"=w2253, "File Name LIN"=w2231, "Pfad Auto Lin"=w2232, "SPAN Idx out"=w2236, "first aktive Komponente"=w2237, w2242, "LIN Filename override"=w2230) -> (w2282:T192)  [unwired: 1 in]
              n1338 = call "Set SPAN Component Tables.vi"("EPA Optionsfeld"=w2238, "Polynom-Ordnung"=w2239, "error in (no error)"=w2276, "Gaskomponente"=w2245, "postprocess"=w2275, "Tabellenref."=w2274) -> ("EPA Ausgangs-Cluster"=w2271:T193, "LIN Ausgangs-Cluster"=w2244:T194, "Daten Aufzeichnen Ausgangs-Cluster"=w2264:T195, "Aktiv EPA"=w2260:T57, "Aktiv LIN"=w2261:bool[])  [unwired: 1 out]
              n1339 = call "Manual Filenames.vi"("Flags Cluster"=w2282, "Zeitstempel"=w2283, "SpanInletClusterArray in"=w2284) -> ("Fehler (Ausgang)"=w2281:errorcluster, "LogInfo-Cluster"=w2248:T196, "Pfad LIN Cluster"=w2240:cluster{"Pfad LIN SPAN":T9, "Pfad LIN":path}, "SpanInletClusterArray out"=w2278:T19[], "Span_Name"=w2241:string, "File Names"=w2279:T197)  [unwired: 1 in, 2 out]
              n1340 = Unbundle(w2240) -> ("Pfad LIN SPAN"=w2234:T9, "Pfad LIN"=w2233:path)
              n1341 = call "get SPAN next active component.vi"("Komponente Idx"=w2237, "SPAN Idx"=w2236, "SpanInletClusterArray in"=w2278) -> ("next aktive Komponente"=w2259:i32, "SPAN Idx out"=w2258:i32)  [unwired: 6 in, 1 out]
              n1342 = Unbundle By Name(w2264) -> ("Ausgabetabelle"=w2263:T53, "Eingabetabelle behandelt"=w2262:string[][])
              n1343 = Unbundle By Name(w2244) -> ("LIN Ausgabetabelle"=w2267:string[][], "XY-Graph"=w2266:cluster{dbl[], dbl[]}[], "Polynomkoeff."=w2265:T198)
              n1344 = Unbundle By Name(w2271) -> ("EPA Ausgabetabelle"=w2270:string[][], "XY-Graph"=w2269:cluster{dbl[], dbl[]}[], "LINVer Auswertung"=w2268:string[][])
              n1345 = call "get SPAN component params EPA LIN.vi"("Index in"=w2235, "LIN Ausgangs-Cluster"=w2244, "Gaskomponente"=w2245, "Component"=w2247) -> ("Component Cluster"=w2246:T199)  [unwired: 4 in, 3 out]
              n1346 = Unbundle By Name(w2279) -> ("LIN TXT Datei Name"=w2280:string)
              n1347 = call "FGV SPAN Verriegelung.vi"("aktion"=Aktion_FGV_SPAN_Verriegelung."setcomp", "Component Cluster"=w2246) -> ()  [unwired: 7 in, 3 out]
              n1348 = case shown="True" w2251 {
                tunnel: w2234 -> [_ w2290]
                tunnel: w2250 -> [_ w2287]
                tunnel: w2252 -> [_ w2289]
                tunnel: [_ w2288] -> _
                tunnel: w2249 -> [_ w2286]
                tunnel: w2248 -> [_ w2285]
                frame False {
                }
                frame True {
                  # "Error Log"
                  n1349 = call "Log SPAN autorun Errors.vi"("Sprachliste"=w2289, "Component Infos"=w2286, "LogInfo-Einstellung-Cluster"=w2287, "LogInfo-Cluster"=w2285, "Pfad LIN"=w2290) -> ("error out"=w2288:errorcluster)  [unwired: 6 in]
                }
              }
            }
            frame True {
              # "automatisch"
              n1350 = call "Postprocess Wrapper active SPAN Comp.vi"("postprocessing"=w2327, "SpanInletClusterArray in"=w2352) -> ("Fehler (Ausgang)"=w2356:errorcluster, "active reprocessing SPAN Component"=w2300:i32, "active reprocessing SPAN"=w2301:i32, "SpanInletClusterArray out"=w2333:T19[])  [unwired: 6 in]
